vi "Self-Test.vi"(8 "error in (no error)":errorcluster, 11 "VISA resource name":refnum<visa-resource-name>) -> (0 "error out":errorcluster, 1 "Last -Test Failed":dbl, 2 "Self-Test Result Message":string, 3 "VISA resource name out":refnum<visa-resource-name>)   [LabVIEW 2019, in "Andeen-Hagerling 2700(400 firmware).lvlib"]
doc: "Performs all (above group 19) diagnostic tests on the internal circuitry of the bridge that require no operator intervention."
uses:
  Andeen-Hagerling 2700(400 firmware).lvlib
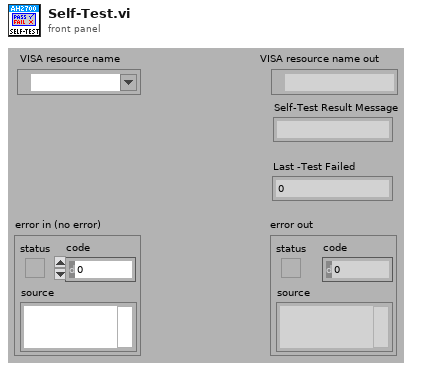
[diagram p1: front panel]
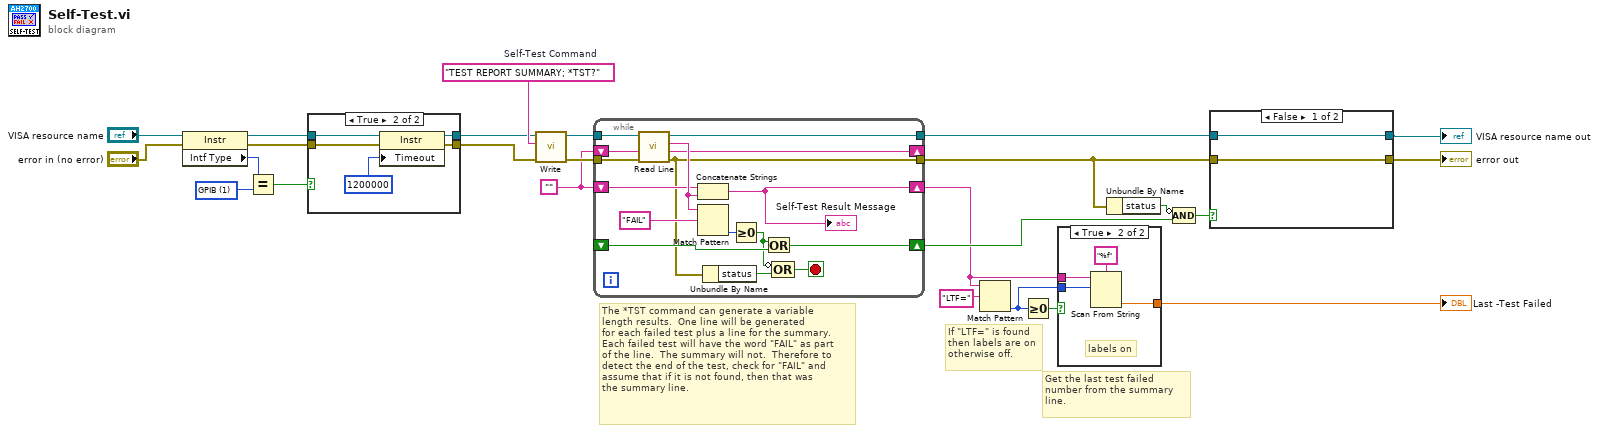
[diagram p0: block diagram]
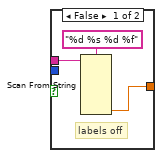
[diagram p3: hidden frame]
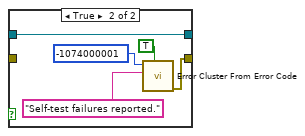
[diagram p4: hidden frame]
diagram:
  w8 = u16 1 items=["GPIB"=1, "VXI"=2, "GPIB-VXI"=3, "Serial"=4, "PXI"=5, "TCPIP"=6, "USB"=7] ("Interface Information:Interface Type")
  w18 = ""
  w21 = "TEST REPORT SUMMARY; *TST?"  # Self-Test Command
  # "If \"LTF=\" is found\nthen labels are on\notherwise off."
  # "Get the last test failed\nnumber from the summary\nline."
  # "The *TST command can generate a variable\nlength results.  One line will be generated\nfor each failed test plus a line for the summary.\nEach failed test will have the word \"FAIL\" as part\nof the line.  The summary will not.  Therefore to\ndetect the end of the test, check for \"FAIL\" and\nassume that if it is not found, then that was\nthe summary line."
  n1 = property class="Instr"(reference="VISA resource name", error in="error in (no error)") -> (reference out=w6:refnum<visa-resource-name>, error out=w4:errorcluster, "Intf Type"=w7:u16)
  n2 = Equal?(x=w7, y=w8) -> (x = y?=w2:bool)
  n3 = case shown="True" w2 {
    tunnel: w6 -> [w27 w32]
    tunnel: [w27 w31] -> w5
    tunnel: w4 -> [w26 w29]
    tunnel: [w26 w28] -> w3
    frame False {
    }
    frame True {
      n4 = property class="Instr"(reference=w32, error in=w29, "Timeout"=u32 1200000 ("General Settings:Timeout Value")) -> (reference out=w31:refnum<visa-resource-name>, error out=w28:errorcluster)
    }
  }
  n5 = call "Write.vi"("error in"=w3, "command"=w21, "VISA resource name"=w5) -> ("error out"=w19:errorcluster, "VISA resource name out"=w20:refnum<visa-resource-name>)  [unwired: 7 in]
  n6 = while {
    shift-right: [w35] -> _
    shift-left: w18 -> [w34]
    tunnel: w20 -> [w42]
    tunnel: w19 -> [w41]
    tunnel: [w43] -> w17
    tunnel: [w39] -> w16
    shift-right: [w33] -> w1
    shift-left: w18 -> [w40]
    shift-right: [w45] -> w15
    shift-left: _ -> [w44]
    stop <- w37 stop-if-true
    n7 = call "Read Line.vi"("error in"=w41, "Previous"=w34, "VISA resource name"=w42) -> ("error out"=w39:errorcluster, "Remaining"=w35:string, "Message"=w48:string, "VISA resource name out"=w43:refnum<visa-resource-name>)  [unwired: 5 in]
    n8 = Concatenate Strings(w40, w48) -> (w33:string)
    "Self-Test Result Message" <- w33
    n9 = Match Pattern(string=w48, regular expression="FAIL") -> (offset past match=w47:i32)  [unwired: 1 in, 3 out]
    n10 = Unbundle By Name(w39) -> ("status"=w38:bool)
    n11 = Greater Or Equal To 0?(x=w47) -> (x >= 0?=w36:bool)
    n12 = Or(x=w36, y=w44) -> (x .or. y?=w45:bool)
    n13 = Compound Arithmetic op=OR(invert w36, w38) -> (w37:bool)
  }
  n14 = Match Pattern(string=w1, regular expression="LTF=") -> (offset past match=w12:i32)  [unwired: 1 in, 3 out]
  n15 = Greater Or Equal To 0?(x=w12) -> (x >= 0?=w13:bool)
  n16 = case shown="True" w13 {
    tunnel: w12 -> [_ w54]
    tunnel: [w49 w53] -> w11
    tunnel: w1 -> [w50 w52]
    frame False {
      # "labels off"
      n17 = Scan From String(format string="%d %s %d %f", input string=w50) -> (output 4=w49:dbl)  [unwired: 9 in, 3 out]
    }
    frame True {
      # "labels on"
      n18 = Scan From String(format string="%f", input string=w52, initial scan location=w54) -> (output 1=w53:dbl)  [unwired: 2 in, 3 out]
    }
  }
  "Last -Test Failed" <- w11
  n19 = Unbundle By Name(w16) -> ("status"=w25:bool)
  n20 = Compound Arithmetic op=AND(invert w25, w15) -> (w24:bool)
  n21 = case shown="False" w24 {
    tunnel: w17 -> [w57 w62]
    tunnel: w16 -> [w56 _]
    tunnel: [w56 w58] -> w22
    tunnel: [w57 w62] -> w23
    frame False {
    }
    frame True {
      n22 = call <vilib>:"Error Cluster From Error Code.vi"("show call chain? (False)"=TRUE, "error message (\"\")"="Self-test failures reported." ("Source (VI Name)"), "error code (0)"=-1074000001 ("Code")) -> ("error out"=w58:errorcluster)  [unwired: 6 in]
    }
  }
  "VISA resource name out" <- w23
  "error out" <- w22
